vi "Config Channel.vi"(4 "Coupling":u16(ring)=1 items=["AC", "DC", "Ground"], 5 "Bandwidth":u16(ring)=2 items=["20 MHz", "250 MHz", "Full"], 6 "Input Impedance":u16(ring) items=["50 Ohm", "1 MOhm"], 7 "error in (no error)":errorcluster, 8 "Vertical Scale":u16(ring)=6 items=["1mV", "2mV", "5mV", "10mV", "20mV", "50mV", "100mV", "200mV", "500mV", "1V", "2V", "5V", "10V"], 9 "Channel":u16(ring) items=["Ch. 01", "Ch 02", "Ch. 03", "Ch. 04"], 10 "Scope Address":refnum<visa-resource-name>) -> (0 "error out":errorcluster, 3 "reference out":refnum<visa-resource-name>)   [LabVIEW 2020]
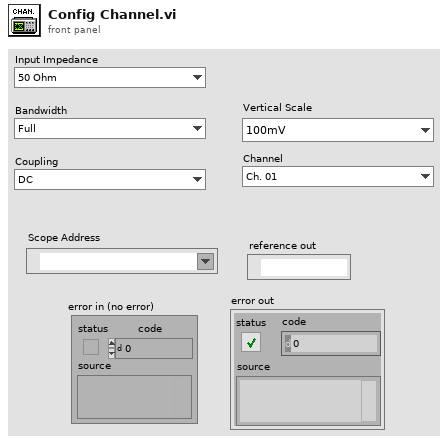
[diagram p1: front panel]
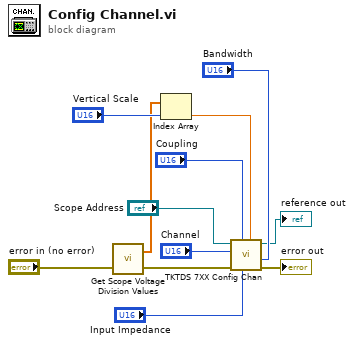
[diagram p0: block diagram]
diagram:
  n1 = call "Get Scope Voltage Division Values.vi"("error in (no error)"="error in (no error)") -> ("error out"=w1:errorcluster, "Volts Per Division Values Array"=w8:dbl[])  [unwired: 1 in]
  n2 = Index Array(array=w8, index="Vertical Scale") -> (element=w9:dbl)
  n3 = call <instrlib>:"TKTDS 7XX Config Chan.vi"("bandwidth (20MHz:0)"="Bandwidth", "scaling (1.0)"=w9, "impedance (50ohms:0)"="Input Impedance", "coupling (DC:1)"="Coupling", "error in (no error)"=w1, "channel to set (ch1:0)"="Channel", "VISA session"="Scope Address") -> ("error out"=→"error out":errorcluster, "dup VISA session"=→"reference out":refnum<visa-resource-name>)  [unwired: 2 in, 1 out]
